vi "HP3488A Close Channels(GPIB).vi"(2 "error in (no error)":errorcluster, 3 "channel addresses":u32[](array[numeric]) min=100, 4 "Device In":cluster{"GPIB":u8, "Address":u8}={"GPIB"=1, "Address"=6} {"Address" min=1 max=31; "GPIB" min=1 max=5}) -> (0 "error out":errorcluster, 1 "Device Out":cluster{"GPIB":u8, "Address":u8}={"GPIB"=1, "Address"=6} {"Address" min=1 max=31; "GPIB" min=1 max=5})   [LabVIEW 2023]
doc: "The HP3488A Close Channels VI is used to simply close one or more relays on the 44470A, 44471A, 44472A, or 44473A option assemblies. It can also be used to 'clear' bits on the 44474A Digital I/O module if it is in default Static Mode #1 or #2."
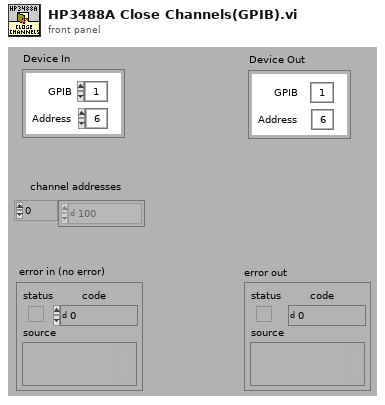
[diagram p1: front panel]
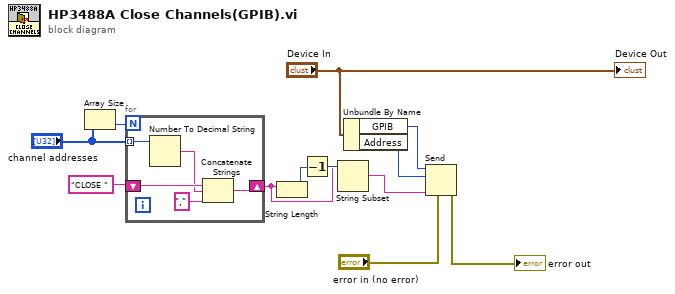
[diagram p0: block diagram]
diagram:
  n1 = Array Size(array="channel addresses") -> (size(s)=w12:i32)
  n2 = for {
    N: w12 -> [_]
    tunnel: "channel addresses" -> [w17] mode=indexing
    shift-right: [w13] -> w9
    shift-left: "CLOSE " -> [w16]
    n3 = Number To Decimal String(number=w17) -> (decimal integer string=w15:string)  [unwired: 1 in]
    n4 = Concatenate Strings(w16, w15, ",") -> (w13:string)
  }
  n5 = String Length(string=w9) -> (length=w11:i32)
  n6 = Decrement(x=w11) -> (x-1=w10:i32)
  n7 = String Subset(string=w9, length (rest)=w10) -> (substring=w3:string)  [unwired: 1 in]
  n8 = Unbundle By Name("Device In") -> ("GPIB"=w2:u8, "Address"=w1:u8)
  n9 = Send(0:w2, 2:w1, 4:"error in (no error)", 5:w3) -> (8:→"error out":errorcluster)  [unwired: 1 in, 2 out]
  "Device Out" <- "Device In"
